vi "数据查询_仪器数据.vi"() -> ()   [LabVIEW 2016]
uses:
  <vilib>/Utility/miscctls.llb/LVPointTypeDef.ctl
  <vilib>/Utility/miscctls.llb/LVRowAndColumnUnsignedTypeDef.ctl
  <userlib>/_OpenG.lib/array/array.llb/Sort 2D Array (String)__ogtk.vi
panel:
  out "布尔":bool
  in  "页":i32 format="第%.0f页"
  in  "每页条数":i32=20
  in  "向后按钮":bool
  in  "向前按钮":bool
  in  "下拉列表":string(xcontrol)
  in  "导出":bool
  out "分钟小时":string(combo)="实时数据"
  out "工作类型":string(combo)="全部数据"
  in  "查询":bool
  in  "结束日期":string="2050/01/01"
  in  "起始日期":string="2010/01/01"
  out "数据表":string[][](table)
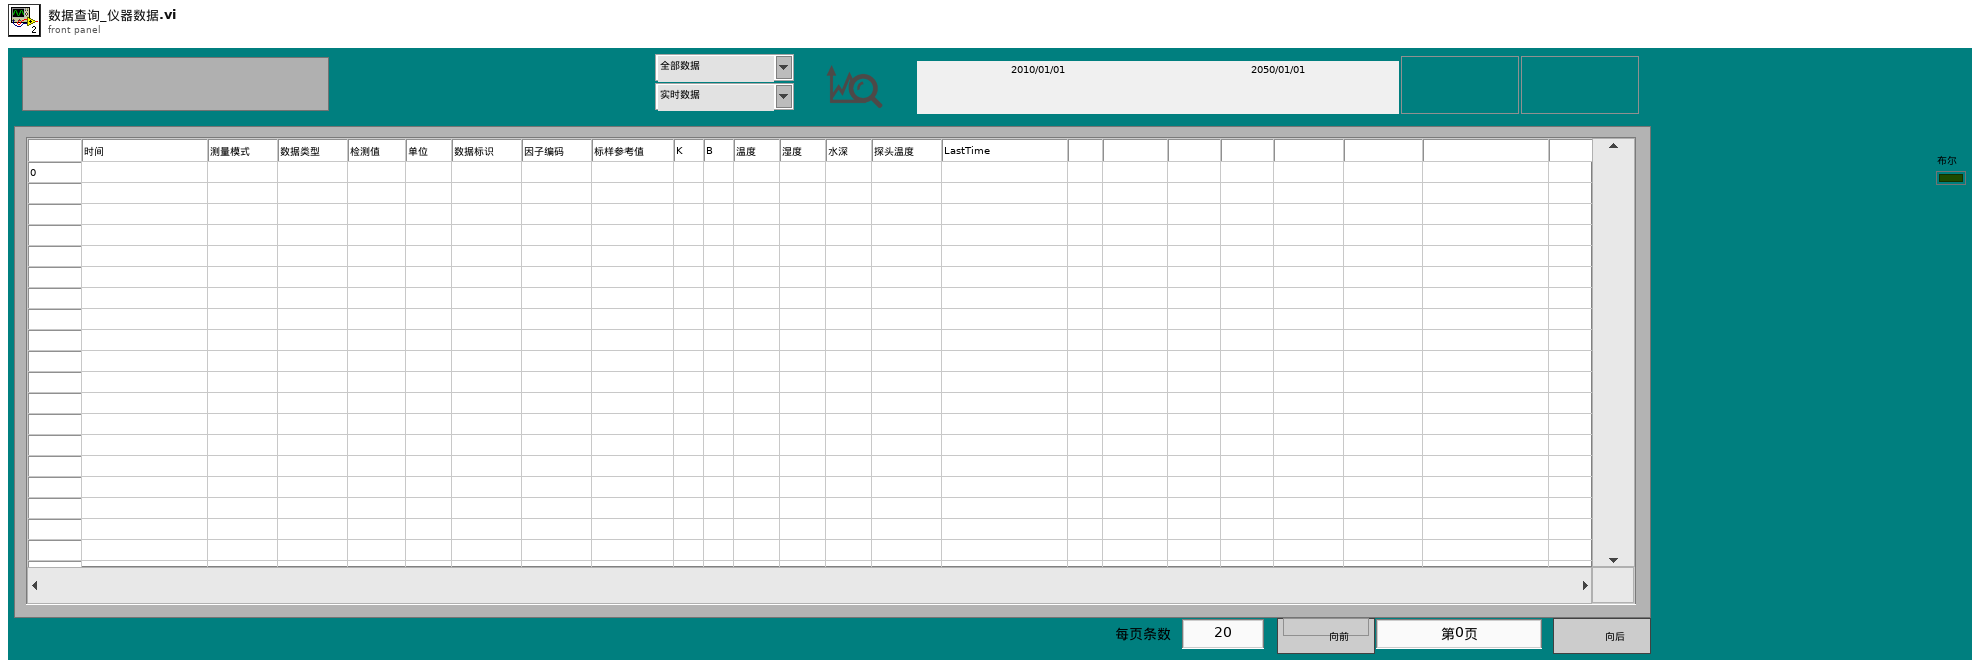
[diagram p1: front panel]
types:
  T1 = typedef "LVPointTypeDef.ctl" = cluster{"Horizontal":i16, "Vertical":i16}
  T2 = typedef "LVDateTimeRec.ctl" = cluster{"秒数的小数部分":dbl, "秒":i32, "分":i32, "时":i32, "日":i32, "月":i32, "年":i32, "天数（周）":i32, "天数（年）":i32, "DST":i32}
  T3 = enum8{"Enabled", "Disabled", "Disabled and Grayed Out"}
  T4 = typedef "LVRowAndColumnUnsignedTypeDef.ctl" = cluster{"Row":u32, "Column":u32}
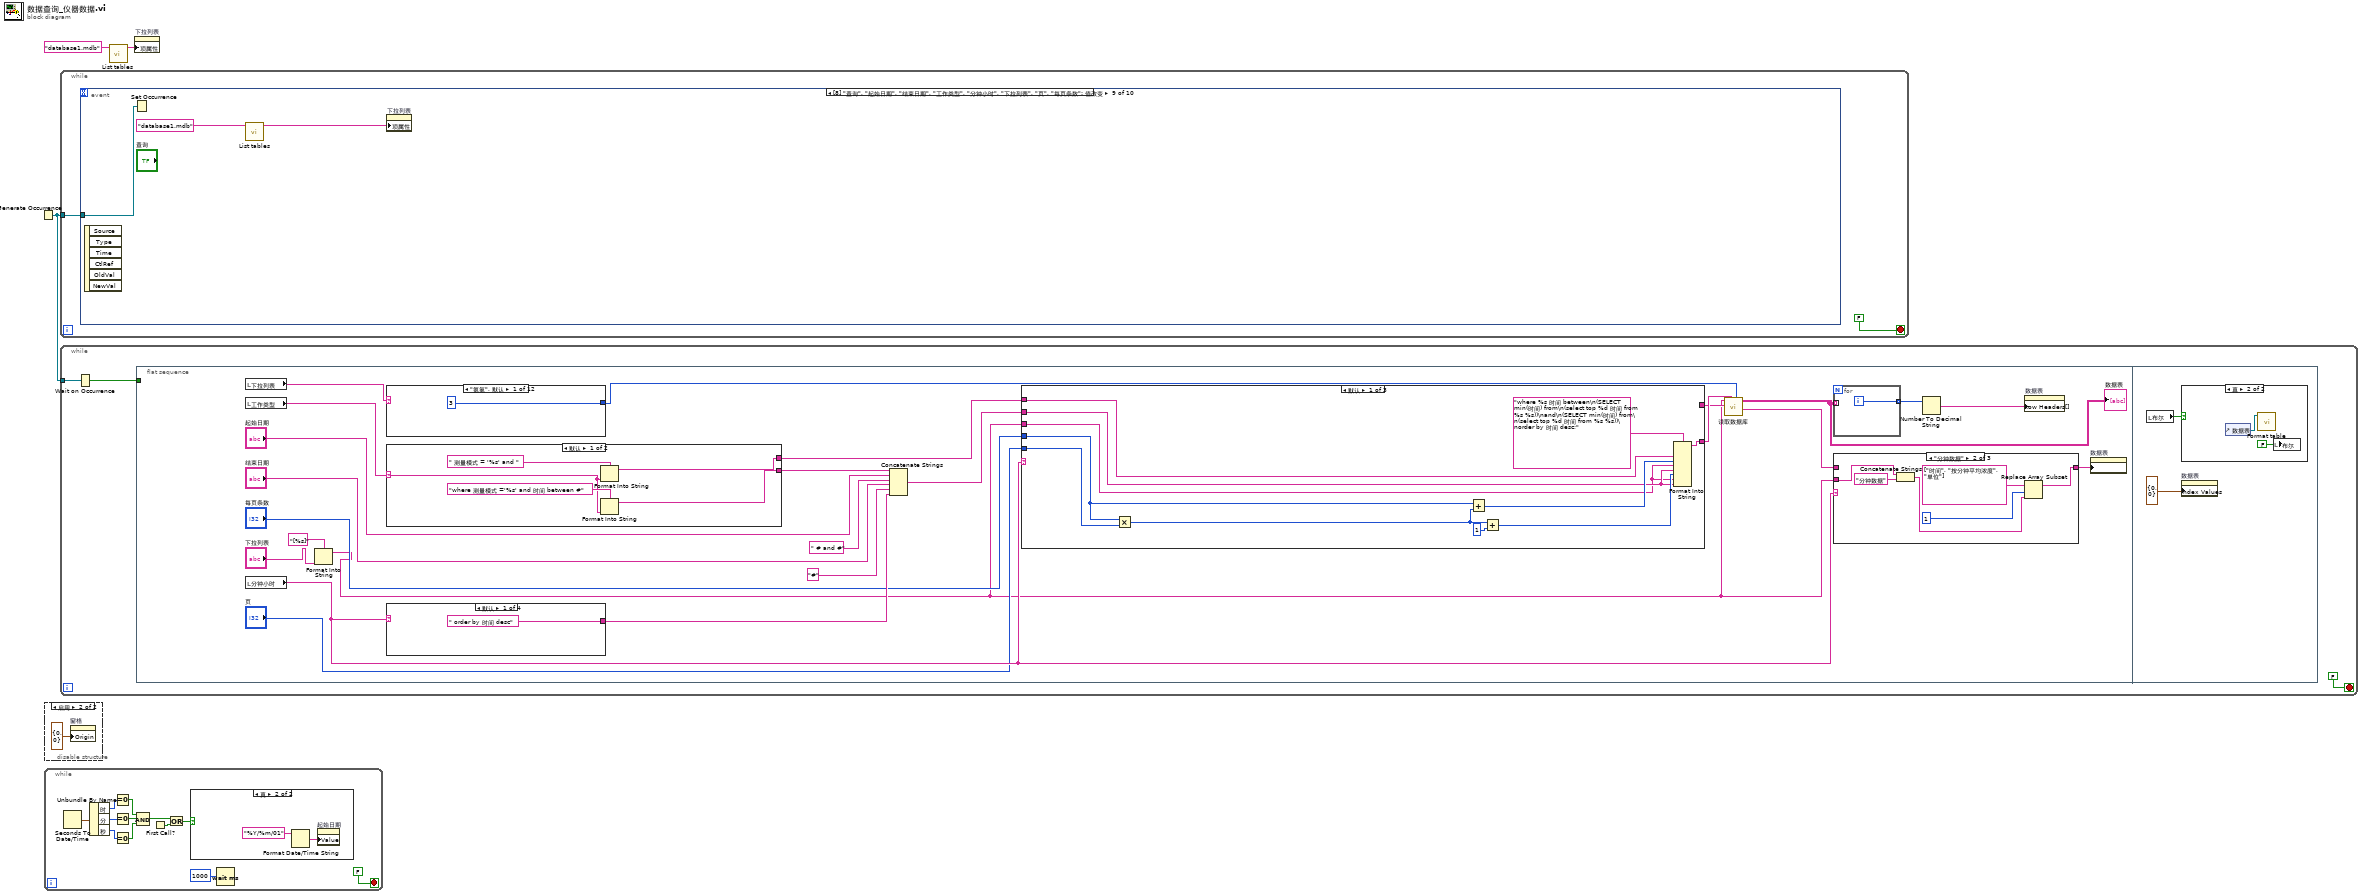
[diagram p0: block diagram]
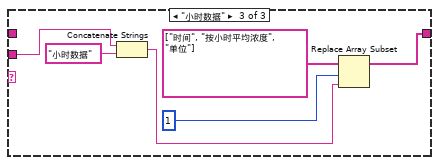
[diagram p3: hidden frame]
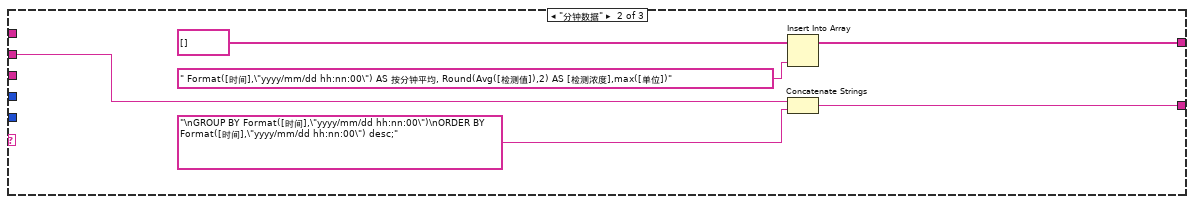
[diagram p7: hidden frame]
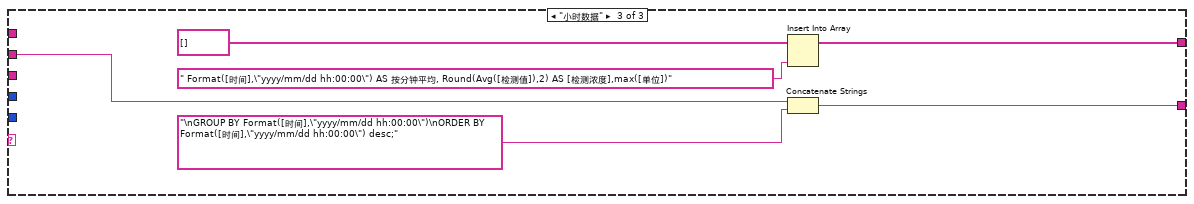
[diagram p8: hidden frame]
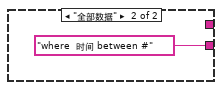
[diagram p9: hidden frame]
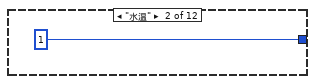
[diagram p10: hidden frame]
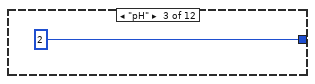
[diagram p11: hidden frame]
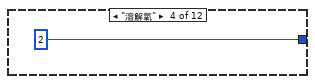
[diagram p12: hidden frame]
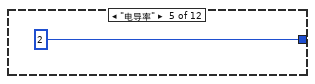
[diagram p13: hidden frame]
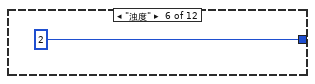
[diagram p14: hidden frame]
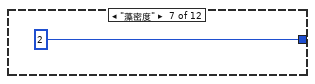
[diagram p15: hidden frame]
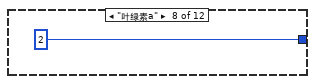
[diagram p16: hidden frame]
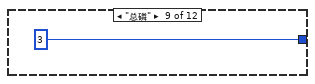
[diagram p17: hidden frame]
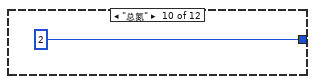
[diagram p18: hidden frame]
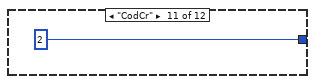
[diagram p19: hidden frame]
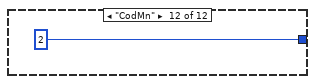
[diagram p20: hidden frame]
diagram:
  n1 = Generate Occurrence() -> (w1:refnum<k4>)
  n2 = disable-structure shown="启用" {
    frame Disabled {
    }
    frame Enabled {
      n3 = property on="窗格" class="Pane"("Origin"=T1 {"Horizontal"=0, "Vertical"=0} ("原点")) -> ()  [unwired: 2 in, 2 out]
    }
  }
  n4 = while {
    stop <- FALSE stop-if-true
    n5 = Seconds To Date/Time() -> (date time rec=w16:T2)  [unwired: 2 in]
    n6 = Unbundle By Name(w16) -> ("时"=w15:i32, "分"=w14:i32, "秒"=w13:i32)
    n7 = Equal To 0?(x=w15) -> (x = 0?=w12:bool)
    n8 = Equal To 0?(x=w14) -> (x = 0?=w11:bool)
    n9 = Equal To 0?(x=w13) -> (x = 0?=w10:bool)
    n10 = Compound Arithmetic op=AND ("复合运算")(w12, w11, w10) -> (w7:bool)
    n11 = First Call?() -> (First Call?: T/F=w5:bool)
    n12 = Or(x=w7, y=w5) -> (x .or. y?=w6:bool)
    n13 = case shown="真" w6 {
      frame False {
      }
      frame True {
        n14 = Format Date/Time String(time format string (%c)="%Y/%m/01" ("时间格式字符串(%c)")) -> (date/time string=w17:string)  [unwired: 2 in]
        n15 = property on="起始日期" class="Str"("Value"=w17) -> ()  [unwired: 2 in, 2 out]
      }
    }
    n16 = Wait (ms)(milliseconds to wait=u32 1000 ("等待时间（毫秒）")) -> ()  [unwired: 1 out]
  }
  n17 = while {
    tunnel: w1 -> [w19]
    stop <- FALSE stop-if-true
    n18 = event shown="[8] \"查询\", \"起始日期\", \"结束日期\", \"工作类型\", \"分钟小时\", \"下拉列表\", \"页\", \"每页条数\": 值改变" {
      selector: _ -> [_ _ _ _ _ _ _ _ _ _]
      dyn-events: _ -> [_ _ _ _ _ _ _ _ _ _]
      timeout: _ -> [_ _ _ _ _ _ _ _ _ _]
      tunnel: w19 -> [_ _ _ _ _ _ _ _ w81 _]
      event Timeout {
        n19 = event-data() -> ()  [unwired: 1 in, 3 out]
      }
      event "查询", "下拉列表": Mouse Down {
        n20 = event-data() -> ()  [unwired: 1 in, 8 out]
        n21 = property on="页" class="DigNum (严格)"("Value"=0 ("页")) -> ()  [unwired: 2 in, 2 out]
        "布尔" <- TRUE ("布尔")
      }
      event "每页条数": Mouse Down {
        n22 = event-data() -> ("CtlRef"=w24:refnum<vi>)  [unwired: 1 in, 7 out]
        n23 = property on="页" class="DigNum (严格)"("Value"=0 ("页")) -> ()  [unwired: 2 in, 2 out]
        n24 = property class="DigNum (严格)"(reference=w24) -> (reference out=w25:refnum<vi>, "Value"=w27:i32)  [unwired: 1 in, 1 out]
        n25 = call "数字键盘.vi"("OldNumber"=w27) -> ("NewNumber"=w26:dbl)
        n26 = property class="DigNum (严格)"(reference=w25, "Val(Sgnl)"=w26) -> ()  [unwired: 1 in, 2 out]
      }
      event "页": Mouse Down {
        n27 = event-data() -> ("CtlRef"=w28:refnum<vi>)  [unwired: 1 in, 7 out]
        n28 = property class="DigNum (严格)"(reference=w28) -> (reference out=w29:refnum<vi>, "Value"=w31:i32)  [unwired: 1 in, 1 out]
        n29 = call "数字键盘.vi"("OldNumber"=w31) -> ("NewNumber"=w30:dbl)
        n30 = property class="DigNum (严格)"(reference=w29, "Val(Sgnl)"=w30) -> ()  [unwired: 1 in, 2 out]
      }
      event "向前按钮": Value Change {
        n31 = event-data() -> ()  [unwired: 1 in, 6 out]
        n32 = property on="页" class="DigNum (严格)"() -> ("Value"=w37:i32)  [unwired: 2 in, 2 out]
        n33 = Decrement(x=w37) -> (x-1=w36:i32)
        n34 = In Range and Coerce(upper limit=9999 ("上限"), x=w36, lower limit=0 ("下限")) -> (coerced(x)=w33:i32, In Range?=w32:bool)
        n35 = case shown="真" w32 {
          tunnel: w33 -> [_ w38]
          frame False {
          }
          frame True {
            n36 = property on="页" class="DigNum (严格)"("Val(Sgnl)"=w38) -> ()  [unwired: 2 in, 2 out]
          }
        }
      }
      event "向后按钮": Value Change {
        n37 = event-data() -> ()  [unwired: 1 in, 6 out]
        n38 = property on="页" class="DigNum (严格)"() -> ("Value"=w43:i32)  [unwired: 2 in, 2 out]
        n39 = Increment(x=w43) -> (x+1=w42:i32)
        n40 = In Range and Coerce(upper limit=u32 9999 ("上限"), x=w42, lower limit=u32 0 ("下限")) -> (coerced(x)=w39:u32)  [unwired: 1 out]
        n41 = property on="页" class="DigNum (严格)"("Val(Sgnl)"=w39) -> ()  [unwired: 2 in, 2 out]
      }
      event "导出": Value Change {
        n42 = event-data() -> ("CtlRef"=w44:refnum<vi>)  [unwired: 1 in, 5 out]
        n43 = property class="Bool"(reference=w44, "DisabledEnum"=T3."Disabled and Grayed Out" ("禁用")) -> (reference out=w48:refnum<vi>, error out=w49:errorcluster)  [unwired: 1 in]
        n44 = flat-sequence {
          tunnel: w49 -> [_]
          tunnel: [w65] -> w47
          tunnel: w48 -> [w65]
          tunnel: "导出" -> [_]
          frame #0 {
            n45 = local read "数据表"() -> (w73:string[][])
            n46 = property on="数据表" class="Tbl (严格)"() -> ("Column Headers[]"=w52:string[])  [unwired: 2 in, 2 out]
            n47 = call "Removable devices detection v8.5.vi"() -> ("Removable"=w62:string[])  [unwired: 4 out]
            n48 = Array Size(array=w52) -> (size(s)=w59:i32)
            n49 = Insert Into Array(array=string[][] [], new element=w52) -> (w51:string[][])  [unwired: 2 in]
            n50 = Index Array(array=w62) -> (element=w61:string)  [unwired: 1 in]
            n51 = call-poly <userlib>:"Sort Array__ogtk.vi"("Column/Row to Sort By"=u32 0, "Sort By in"=enum16{"row", "column"}."column", "Order"=enum16{"ascending", "descending"}."ascending", "Array in"=w73) -> ("Sorted Array out"=w72:string[][])  [unwired: 4 in, 3 out]
            n52 = String To Path(string=w61) -> (path=w60:path)
            n53 = Greater Or Equal?(x=w59, y=5) -> (x >= y?=w57:bool)
            n54 = Select(t=3 ("禁用的索引 (列)"), s=w57, f=1) -> (s? t:f=w55:i32)
            n55 = Index Array(array=w72, index (col)=w55) -> (element=w68:string[])  [unwired: 1 in]
            n56 = Get Date/Time In Seconds() -> (seconds since 1Jan1904=w74:timestamp)
            n57 = local read "下拉列表"() -> (w66:string)
            n58 = Fract/Exp String To Number(string=w68) -> (number=w67:dbl[])  [unwired: 3 in, 1 out]
            n59 = call "MS Office Report"("Path to Save Report"=w60, "导出日期"=w74, "监测参数"=w66, "数据输入"=w72, "图表输入"=w67, "字段定义"=w51) -> ("error out"=w64:errorcluster)  [unwired: 20 in, 1 out]
            n60 = case shown="错误" w64 {
              tunnel: ["导出成功" ("消息") "导出失败" ("消息")] -> w63
              frame No Error {
              }
              frame Error {
              }
            }
            n61 = One Button Dialog(message=w63) -> ()  [unwired: 1 in, 1 out]
          }
        }
        n62 = property class="Bool"(reference=w47, "DisabledEnum"=T3."Enabled" ("禁用")) -> ()  [unwired: 1 in, 2 out]
      }
      event "起始日期", "结束日期": Mouse Down {
        n63 = event-data() -> ("CtlRef"=w80:refnum<vi>)  [unwired: 1 in, 7 out]
        n64 = property class="Str"(reference=w80) -> (reference out=w78:refnum<vi>, "Value"=w79:string)  [unwired: 1 in, 1 out]
        n65 = call "日期键盘.vi"("原值"=w79) -> ("x+y"=w77:string)  [unwired: 10 in]
        n66 = property class="Str"(reference=w78, "Val(Sgnl)"=w77) -> ()  [unwired: 1 in, 2 out]
      }
      event "查询", "起始日期", "结束日期", "工作类型", "分钟小时", "下拉列表", "页", "每页条数": Value Change {
        n67 = event-data() -> ()  [unwired: 1 in, 6 out]
        n68 = Set Occurrence(w81) -> ()
        n69 = call "List tables.vi"("database"="database1.mdb") -> ("tables"=w82:string[])  [unwired: 9 in, 1 out]
        n70 = property on="下拉列表" class="下拉列表 (严格)"("项属性"=w82) -> ()  [unwired: 2 in, 2 out]
      }
      event "工作类型", "分钟小时": Mouse Down {
        n71 = event-data() -> ()  [unwired: 1 in, 8 out]
        n72 = call "数据查询筛选.vi"() -> ("分钟小时"=→"分钟小时":string, "工作类型"=w84:string)  [unwired: 10 in]
        n73 = property on="工作类型" class="CmbBox"("Val(Sgnl)"=w84) -> ()  [unwired: 2 in, 2 out]
      }
    }
  }
  n74 = while {
    tunnel: w1 -> [w87]
    stop <- FALSE stop-if-true
    n75 = Wait on Occurrence(2:w87) -> (0:w86:bool)  [unwired: 2 in]
    n76 = flat-sequence {
      tunnel: w86 -> [_]
      frame #0 {
        n77 = local read "下拉列表"() -> (w105:string)
        n78 = local read "工作类型"() -> (w103:string)
        n79 = local read "分钟小时"() -> (w97:string)
        n80 = Format Into String(format string="[%s]" ("格式字符串"), "下拉列表") -> (resulting string=w89:string)  [unwired: 2 in, 1 out]
        n81 = case shown="\"氨氮\", 默认" w105 {
          tunnel: [i16 3 ("精度(6)") i16 1 ("精度(6)") i16 2 ("精度(6)") i16 2 ("精度(6)") i16 2 ("精度(6)") i16 2 ("精度(6)") i16 2 ("精度(6)") i16 2 ("精度(6)") i16 3 ("精度(6)") i16 2 ("精度(6)") i16 2 ("精度(6)") i16 2 ("精度(6)")] -> w104
          frame "氨氮", Default {
          }
          frame "水温" {
          }
          frame "pH" {
          }
          frame "溶解氧" {
          }
          frame "电导率" {
          }
          frame "浊度" {
          }
          frame "藻密度" {
          }
          frame "叶绿素a" {
          }
          frame "总磷" {
          }
          frame "总氮" {
          }
          frame "CodCr" {
          }
          frame "CodMn" {
          }
        }
        n82 = case shown="默认" w103 {
          selector: w103 -> [w151 _]
          tunnel: [w153 "where  时间 between #" ("condition")] -> w102
          tunnel: [w150 _] -> w92
          frame Default {
            n83 = Format Into String(format string=" 测量模式 = '%s' and " ("condition"), w151) -> (resulting string=w150:string)  [unwired: 2 in, 1 out]
            n84 = Format Into String(format string="where 测量模式 ='%s' and 时间 between #" ("condition"), w151) -> (resulting string=w153:string)  [unwired: 2 in, 1 out]
          }
          frame "全部数据" {
          }
        }
        n85 = case shown="默认" w97 {
          tunnel: [" order by 时间 desc" ("字符串") _ _ _] -> w101
          frame Default {
          }
          frame "分钟数据" {
          }
          frame "小时数据" {
          }
          frame "真" {
          }
        }
        n86 = Concatenate Strings(w102, "起始日期", " # and #" ("condition"), "结束日期", "#" ("condition"), w101) -> (w100:string)
        n87 = case shown="默认" w97 {
          tunnel: [_ w142 w144] -> w98
          tunnel: w100 -> [w129 w140 w146]
          tunnel: [w132 w139 w145] -> w99
          tunnel: w89 -> [w128 _ _]
          tunnel: "每页条数" -> [w131 _ _]
          tunnel: "页" -> [w130 _ _]
          tunnel: w92 -> [w127 _ _]
          frame Default {
            n88 = Multiply(x=w131, y=w130) -> (x*y=w136:i32)
            n89 = Add(x=w131, y=w136) -> (x+y=w134:i32)
            n90 = Add(x=w136, y=u32 1) -> (x+y=w133:u32)
            n91 = Format Into String(format string="where %s 时间 between\n(SELECT min(时间) from\n(select top %d 时间 from %s %s))\nand\n(SELECT min(时间) from\n(select top %d 时间 from %s %s))\norder by 时间 desc;" ("格式字符串"), w127, w134, w128, w129, w133, w128, w129) -> (resulting string=w132:string)  [unwired: 2 in, 1 out]
          }
          frame "分钟数据" {
            n92 = Insert Into Array(array=string[] [] ("显示项"), new element=" Format([时间],\"yyyy/mm/dd hh:nn:00\") AS 按分钟平均, Round(Avg([检测值]),2) AS [检测浓度],max([单位])" ("新元素/子数组")) -> (w142:string[])  [unwired: 1 in]
            n93 = Concatenate Strings(w140, "\nGROUP BY Format([时间],\"yyyy/mm/dd hh:nn:00\")\nORDER BY Format([时间],\"yyyy/mm/dd hh:nn:00\") desc;" ("字符串")) -> (w139:string)
          }
          frame "小时数据" {
            n94 = Insert Into Array(array=string[] [] ("显示项"), new element=" Format([时间],\"yyyy/mm/dd hh:00:00\") AS 按分钟平均, Round(Avg([检测值]),2) AS [检测浓度],max([单位])" ("新元素/子数组")) -> (w144:string[])  [unwired: 1 in]
            n95 = Concatenate Strings(w146, "\nGROUP BY Format([时间],\"yyyy/mm/dd hh:00:00\")\nORDER BY Format([时间],\"yyyy/mm/dd hh:00:00\") desc;" ("字符串")) -> (w145:string)
          }
        }
        n96 = call "读取数据库.vi"("精度(6)"=w104, "condition"=w99, "显示项"=w98, "组合框"=w89) -> ("columns"=w96:string[], "表格"=w108:string[][])  [unwired: 4 in, 2 out]
        "数据表" <- w108
        n97 = for {
          tunnel: w108 -> [_] mode=indexing
          tunnel: [w168] -> w107 mode=indexing
          i -> [w168]
        }
        n98 = case shown="\"分钟数据\"" w97 {
          tunnel: w96 -> [w113 _ _]
          tunnel: [w113 w117 w121] -> w95
          tunnel: w89 -> [_ w116 w122]
          frame Default {
          }
          frame "分钟数据" {
            n99 = Concatenate Strings(w116, "分钟数据" ("字符串")) -> (w114:string)
            n100 = Replace Array Subset(array=string[] ["时间", "按分钟平均浓度", "单位"] ("columns"), new element=w114, index=1 ("索引")) -> (w117:string[])
          }
          frame "小时数据" {
            n101 = Concatenate Strings(w122, "小时数据" ("字符串")) -> (w123:string)
            n102 = Replace Array Subset(array=string[] ["时间", "按小时平均浓度", "单位"] ("columns"), new element=w123, index=1 ("索引")) -> (w121:string[])
          }
        }
        n103 = Number To Decimal String(number=w107) -> (decimal integer string=w106:string[])  [unwired: 1 in]
        n104 = property on="数据表" class="Tbl (严格)"("Row Headers[]"=w106) -> ()  [unwired: 2 in, 2 out]
        n105 = property on="数据表" class="Tbl (严格)"("Column Headers[]"=w95) -> ()  [unwired: 2 in, 2 out]
      }
      frame #1 {
        n106 = local read "布尔"() -> (w169:bool)
        n107 = case shown="真" w169 {
          frame False {
          }
          frame True {
            n108 = control-ref of="数据表"() -> (w172:refnum<vi>)
            n109 = call "Format table.vi"("Table输入"=w172) -> ()  [unwired: 11 in]
            n110 = local write "布尔"(FALSE ("布尔")) -> ()
          }
        }
        n111 = property on="数据表" class="Tbl (严格)"("Index Values"=T4 {"Row"=0, "Column"=0} ("索引值")) -> ()  [unwired: 2 in, 2 out]
      }
    }
  }
  n112 = call "List tables.vi"("database"="database1.mdb") -> ("tables"=w2:string[])  [unwired: 9 in, 1 out]
  n113 = property on="下拉列表" class="下拉列表 (严格)"("项属性"=w2) -> ()  [unwired: 2 in, 2 out]
